vi "Binary to Nominal.vi"(0 "Target Type":T1(ring), 5 "Channel Calibration":cluster{"LSB Weight":u32, "Offset":i32}, 9 "Binary Value":i16) -> (4 "Units":enum8{"mA", "V", "V/V", "Ohms"}(ring), 10 "Nominal Value":dbl)   [LabVIEW 2020]
doc: "Converts a binary value to its nominal value equivalent.."
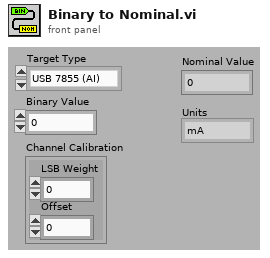
[diagram p1: front panel]
types:
  T1 = enum16{"USB 7855 (AI)", "USB 7855 (AO)", "USB 7855 OEM (AI)", "USB 7855 OEM (AO)", "USB 7856  (AI)", "USB 7856 (AO)", "USB 7856 OEM (AI)", "USB 7856 OEM (AO)"}
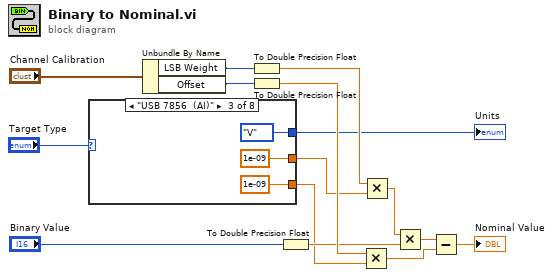
[diagram p0: block diagram]
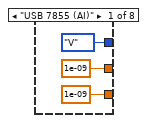
[diagram p2: hidden frame]
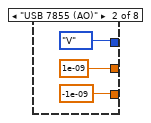
[diagram p3: hidden frame]
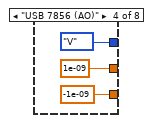
[diagram p4: hidden frame]
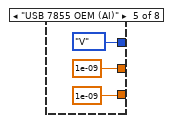
[diagram p5: hidden frame]
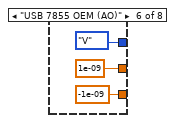
[diagram p6: hidden frame]
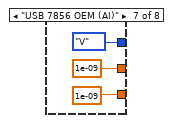
[diagram p7: hidden frame]
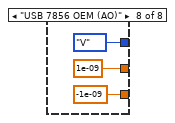
[diagram p8: hidden frame]
diagram:
  n1 = case shown="\"USB 7856  (AI)\"" "Target Type" {
    tunnel: [1e-09 ("y") 1e-09 ("y") 1e-09 ("y") 1e-09 ("y") 1e-09 ("y") 1e-09 ("y") 1e-09 ("y") 1e-09 ("y")] -> w2
    tunnel: [1e-09 ("y") -1e-09 ("y") 1e-09 ("y") -1e-09 ("y") 1e-09 ("y") -1e-09 ("y") 1e-09 ("y") -1e-09 ("y")] -> w3
    tunnel: [enum8{"mA", "V", "V/V", "Ohms"}."V" ("Units") enum8{"mA", "V", "V/V", "Ohms"}."V" ("Units") enum8{"mA", "V", "V/V", "Ohms"}."V" ("Units") enum8{"mA", "V", "V/V", "Ohms"}."V" ("Units") enum8{"mA", "V", "V/V", "Ohms"}."V" ("Units") enum8{"mA", "V", "V/V", "Ohms"}."V" ("Units") enum8{"mA", "V", "V/V", "Ohms"}."V" ("Units") enum8{"mA", "V", "V/V", "Ohms"}."V" ("Units")] -> w1
    frame "USB 7855 (AI)" {
    }
    frame "USB 7855 (AO)" {
    }
    frame "USB 7856  (AI)" {
    }
    frame "USB 7856 (AO)" {
    }
    frame "USB 7855 OEM (AI)" {
    }
    frame "USB 7855 OEM (AO)" {
    }
    frame "USB 7856 OEM (AI)" {
    }
    frame "USB 7856 OEM (AO)" {
    }
  }
  "Units" <- w1
  n2 = Unbundle By Name("Channel Calibration") -> ("LSB Weight"=w14:u32, "Offset"=w12:i32)
  n3 = To Double Precision Float(number=w14) -> (double precision float=w7:dbl)
  n4 = To Double Precision Float(number=w12) -> (double precision float=w8:dbl)
  n5 = To Double Precision Float(number="Binary Value") -> (double precision float=w6:dbl)
  n6 = Multiply(x=w8, y=w3) -> (x*y=w10:dbl)
  n7 = Multiply(x=w7, y=w2) -> (x*y=w13:dbl)
  n8 = Multiply(x=w13, y=w6) -> (x*y=w11:dbl)
  n9 = Subtract(x=w11, y=w10) -> (x-y=→"Nominal Value":dbl)
